vi "Strtok, Four Strings.vi"(0 "delimiters (\\s\\t\\r\\n=)":string=" \t\r\n=", 1 "offset":i32, 2 "input string":string="2.3 745") -> (3 "token 4":string, 4 "token 3":string, 5 "token 2":string, 6 "token 1":string)   [LabVIEW 2010]
doc: "Scans the input string, starting at offset, for tokens, and outputs four double precision floating point values."
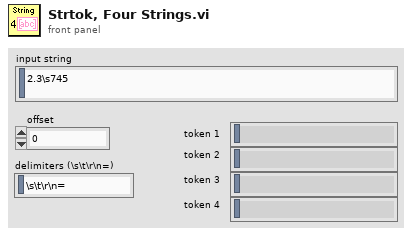
[diagram p1: front panel]
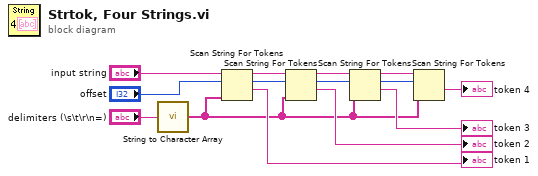
[diagram p0: block diagram]
diagram:
  n1 = call "String to Character Array.vi"("input string"="delimiters (\\s\\t\\r\\n=)") -> ("character array"=w3:string[])
  n2 = Scan String For Tokens(6:w3, 8:"offset", 9:"input string") -> (1:→"token 1":string, 2:w12:i32, 3:w13:string)  [unwired: 3 in, 1 out]
  n3 = Scan String For Tokens(6:w3, 8:w12, 9:w13) -> (1:→"token 2":string, 2:w8:i32, 3:w10:string)  [unwired: 3 in, 1 out]
  n4 = Scan String For Tokens(6:w3, 8:w8, 9:w10) -> (1:→"token 3":string, 2:w7:i32, 3:w9:string)  [unwired: 3 in, 1 out]
  n5 = Scan String For Tokens(6:w3, 8:w7, 9:w9) -> (1:→"token 4":string)  [unwired: 3 in, 3 out]
